vi "Extract8BitImage.vi"(2 "Flip?":bool, 3 "Image in":T1 {"Dialogs" format="%.0b"}) -> (0 "Intensity Graph":u8[][](graph), 1 "Image out":T1 {"Dialogs" format="%.0b"})   [LabVIEW 2024]
doc: "This VI converts an 8 bit image into a 2-dimensional array \nof rows and columns (e.g. 320 columns and 240 rows).\n\nModifier: \nFlip: If true, this will flip the image so that the image looks right in the Intensity graph (element 0,0 in a picture is the upper left corner but in a graph is in the lower left). Default is False."
uses:
  <userlib>/ImageProcessing/QTLIB_2595_LV86/QT_Image.ctl
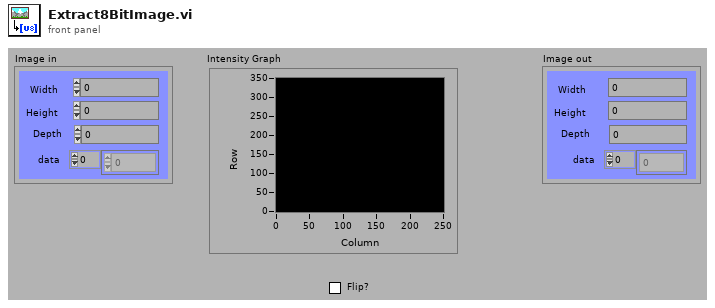
[diagram p1: front panel]
types:
  T1 = typedef "QT_Image.ctl" = cluster{"Width":i32, "Height":i32, "Depth":i32, "data":u8[], "Compressed data":u8[], "Color table":u32[], "Duration":i32, "Options":i32, "Timestamp":i32, "ID":i32, "Reserved":i32, "Dialogs":u32}
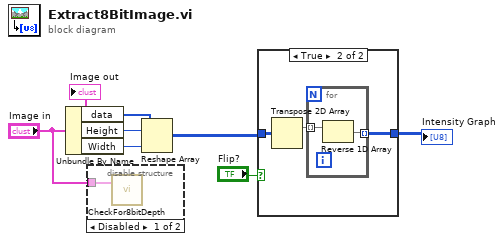
[diagram p0: block diagram]
diagram:
  n1 = Unbundle By Name("Image in") -> ("data"=w5:u8[], "Height"=w7:i32, "Width"=w6:i32)
  n2 = disable-structure shown="Disabled" {
    disable-tunnel: "Image in" -> [w8 _]
    frame Disabled {
      n3 = call <userlib>:"CheckFor8bitDepth.vi"("Image in"=w8) -> ()  [unwired: 2 in, 1 out]
    }
    frame Enabled {
    }
  }
  n4 = Reshape Array(w5, w7, w6) -> (w3:u8[][])
  n5 = case shown="True" "Flip?" {
    tunnel: w3 -> [w9 w12]
    tunnel: [w9 w10] -> w2
    frame False {
    }
    frame True {
      n6 = Transpose 2D Array(2D array=w12) -> (transposed array=w11:u8[][])
      n7 = for {
        tunnel: w11 -> [w14] mode=indexing
        tunnel: [w13] -> w10 mode=indexing
        n8 = Reverse 1D Array(array=w14) -> (reversed array=w13:u8[])
      }
    }
  }
  "Intensity Graph" <- w2
  "Image out" <- "Image in"
